vi "update methane inflow.vi"(8 "error in (no error)":errorcluster, 10 "methane_specfile":string, 11 "outflow_infile":string) -> (0 "error out":errorcluster)   [LabVIEW 2019, in "libFileFunctions.lvlib"]
doc: "void update_methane_inflow(const char* outflow_infile, const char* methane_specfile);"
uses:
  libFileFunctions.lvlib
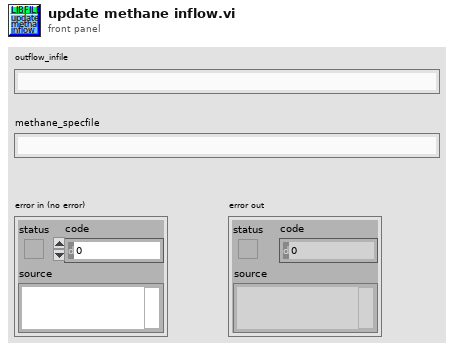
[diagram p1: front panel]
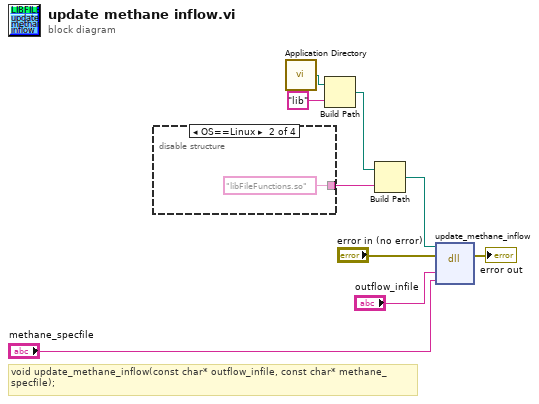
[diagram p0: block diagram]
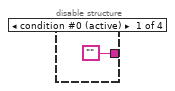
[diagram p2: hidden frame]
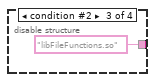
[diagram p3: hidden frame]
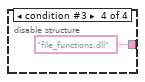
[diagram p4: hidden frame]
diagram:
  # "void update_methane_inflow(const char* outflow_infile, const char* methane_specfile);"
  n1 = disable-structure shown="OS==Linux" {
    disable-tunnel: ["" "libFileFunctions.so" ("name or relative path") "libFileFunctions.so" ("name or relative path") "file_functions.dll" ("name or relative path")] -> w2
    frame condition #0 (active) {
    }
    frame condition #1 {
    }
    frame condition #2 {
    }
    frame condition #3 {
    }
  }
  n2 = call <vilib>:"Application Directory.vi"() -> ("Application Directory"=w5:path)
  n3 = Build Path(base path=w5, name or relative path="lib") -> (appended path=w3:path)
  n4 = Build Path(base path=w3, name or relative path=w2) -> (appended path=w1:path)
  n5 = dll-call lib="home/paul/Schreibtisch/Biogas_plant_setup/LabView/lib/libFileFunctions/libFileFunctions.*" fn="update_methane_inflow"(path in=w1, error in="error in (no error)", "outflow_infile"="outflow_infile", "methane_specfile"="methane_specfile") -> (error out=→"error out":errorcluster)  [unwired: 4 in, 1 out]
